vi "Delete Channel.vi"(8 "error in (no error)":errorcluster, 9 "Index":i32, 11 "SignalManager in":refnum<class "SignalManager.lvclass">) -> (0 "error out":errorcluster, 3 "SignalManager out":refnum<class "SignalManager.lvclass">)   [LabVIEW 2015, in "SignalManager.lvclass"]
uses:
  SignalManager.lvclass
  SignalManager.lvclass/SignalManager.ctl
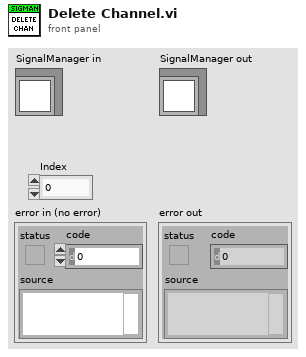
[diagram p1: front panel]
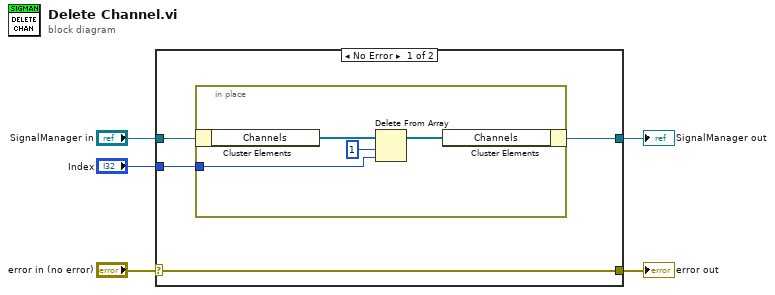
[diagram p0: block diagram]
diagram:
  n1 = case shown="No Error" "error in (no error)" {
    selector: "error in (no error)" -> [w9 w15]
    tunnel: [w9 w15] -> w4
    tunnel: [w7 w14] -> w2
    tunnel: "SignalManager in" -> [w8 w14]
    tunnel: "Index" -> [w6 _]
    frame No Error {
      n2 = in-place {
        in-place-border: w6 -> [w11]
        n3 = in-place-cluster #1(w8) -> ("Channels"=w13:refnum<class "Channel.lvclass">[])
        n4 = Delete From Array(array=w13, length=1, index=w11) -> (array with subset deleted=w12:refnum<class "Channel.lvclass">[])  [unwired: 1 out]
        n5 = in-place-cluster #1("Channels"=w12) -> (w7:refnum<class "SignalManager.lvclass">)
      }
    }
    frame Error {
    }
  }
  "error out" <- w4
  "SignalManager out" <- w2
